vi "Uniform (Discrete) CDF.vi"(10 "n":i32=100, 11 "x":dbl=1.0) -> (0 "error":i32, 3 "cdf(x)":dbl=0.01)   [LabVIEW 2020, in "NI_Gmath.lvlib"]
doc: "Computes the discrete cumulative distribution function (CDF), or the probability that the random variate X, where X describes the selected distribution type, takes on a value less than or equal to <B>x</B>. You must manually select the polymorphic instance to use."
uses:
  NI_Gmath.lvlib
  st_error_code.ctl
panel:
  # "Uniform (Discrete) CDF"
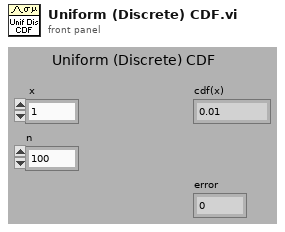
[diagram p1: front panel]
types:
  T1 = typedef "NI_Gmath.lvlib/st_error_code.ctl" = i32
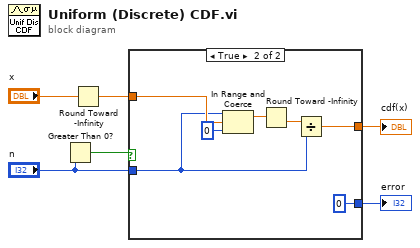
[diagram p0: block diagram]
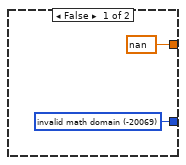
[diagram p2: hidden frame]
diagram:
  n1 = Greater Than 0?(x="n") -> (x > 0?=w4:bool)
  n2 = Round Toward -Infinity(1:"x") -> (0:w1:dbl)
  n3 = case shown="True" w4 {
    tunnel: [nan w10] -> w6
    tunnel: [w7 0 ("invalid math domain")] -> w5
    tunnel: w1 -> [_ w14]
    tunnel: "n" -> [_ w12]
    frame False {
      w7 = T1 -20069 items=["invalid math domain"=-20069, "Fourier interpolation size m >= n"=-20070, "empty array"=-20003] ("stat interp error code")
    }
    frame True {
      n4 = In Range and Coerce(upper limit=w12, x=w14, lower limit=0) -> (coerced(x)=w13:dbl)  [unwired: 1 out]
      n5 = Round Toward -Infinity(1:w13) -> (0:w11:dbl)
      n6 = Divide(x=w11, y=w12) -> (x/y=w10:dbl)
    }
  }
  "cdf(x)" <- w6
  "error" <- w5
